vi "createLateralPressurePIDParametersFrame.vi"(8 "error in (no error)":errorcluster, 9 "TriggerIRQ":bool, 10 "WaitForTrigger":bool, 11 "FAILC in":refnum<class "FAILC.lvclass">) -> (0 "error out":errorcluster, 2 "Frame":T1 {"Data" format="%02x"}, 3 "FAILC out":refnum<class "FAILC.lvclass">)   [LabVIEW 2016, in "RTFAILC.lvlib" / "FAILC.lvclass"]
uses:
  FAILC.lvclass
  Common_RT_Modbus/DataTypes/Frame.ctl
  FAILC.lvclass/FAILC.ctl
  Common_RT_Modbus/RTModbus.lvlib
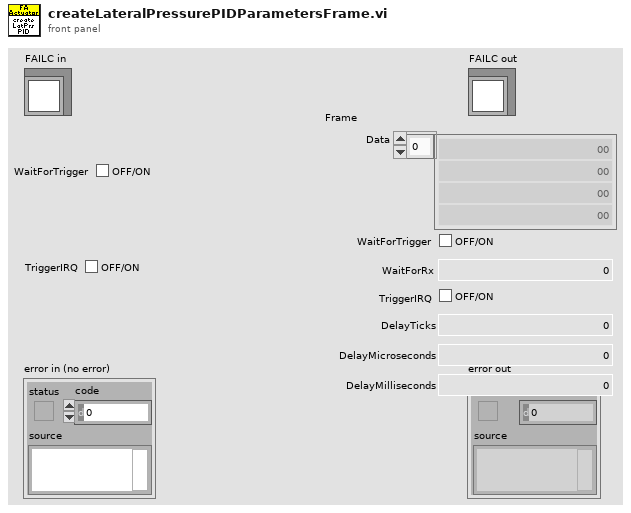
[diagram p1: front panel]
types:
  T1 = typedef "RTModbus.lvlib/Frame.ctl" = cluster{"Data":u8[], "WaitForTrigger":bool, "WaitForRx":u16, "TriggerIRQ":bool, "DelayTicks":u16, "DelayMicroseconds":u16, "DelayMilliseconds":u16}
  T2 = typedef "RTFAILC.lvlib/FAPID.ctl" = cluster{"Kp":sgl, "Ki":sgl, "Kd":sgl, "Kf":sgl}
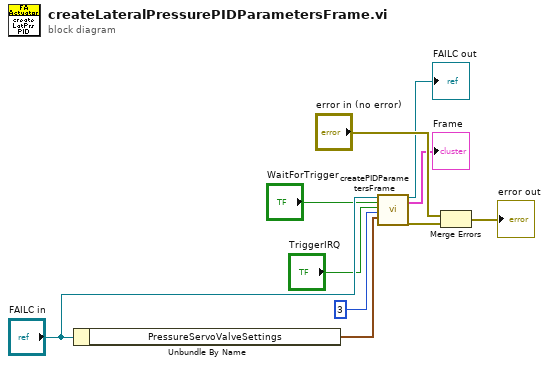
[diagram p0: block diagram]
diagram:
  n1 = Unbundle By Name("FAILC in") -> ("PressureServoValveSettings"=w3:T2)
  n2 = call "createPIDParametersFrame.vi"("FAILC in"="FAILC in", "WaitForTrigger"="WaitForTrigger", "TriggerIRQ"="TriggerIRQ", "PIDNumber"=u8 3, "FAPID"=w3) -> ("FAILC out"=→"FAILC out":refnum<class "FAILC.lvclass">, "Frame"=→"Frame":T1, "error out"=w2:errorcluster)  [unwired: 12 in]
  n3 = Merge Errors("error in (no error)", w2) -> (→"error out":errorcluster)
